vi "Clean Up Structures.vi"(8 "error in (no error)":errorcluster, 11 "Block Diagram in":refnum<class "Block Diagram.lvclass">) -> (0 "error out":errorcluster, 3 "Block Diagram out":refnum<class "Block Diagram.lvclass">)   [LabVIEW 2015, in "Block Diagram.lvclass"]
uses:
  Block Diagram.lvclass
  Block Diagram.lvclass/Block Diagram.ctl
  Structures/Structures.lvclass
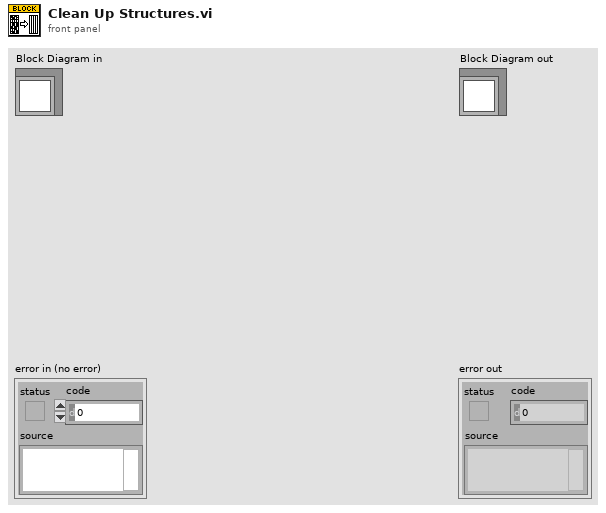
[diagram p1: front panel]
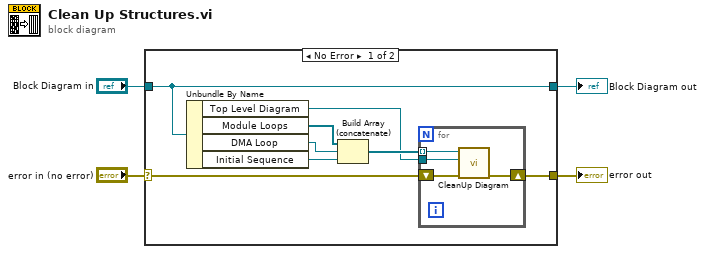
[diagram p0: block diagram]
diagram:
  n1 = case shown="No Error" "error in (no error)" {
    selector: "error in (no error)" -> [w11 w18]
    tunnel: [w5 w18] -> w3
    tunnel: [w12 w17] -> w1
    tunnel: "Block Diagram in" -> [w12 w17]
    frame No Error {
      n2 = Unbundle By Name(w12) -> ("Top Level Diagram"=w7:refnum<vi>, "Module Loops"=w9:refnum<class "Module Loop.lvclass">[], "DMA Loop"=w10:refnum<class "DMA Loop.lvclass">, "Initial Sequence"=w6:refnum<class "Main Sequence.lvclass">)
      n3 = Build Array (concatenate)(w9, w10, w6) -> (w8:refnum<class "Structures.lvclass">[])
      n4 = for {
        tunnel: w8 -> [w16] mode=indexing
        tunnel: w7 -> [w15]
        shift-right: [w13] -> w5
        shift-left: w11 -> [w14]
        n5 = call-dynamic "CleanUp Diagram.vi"("error in (no error)"=w14, "Top Level Diagram"=w15, "Structures in"=w16) -> ("error out"=w13:errorcluster)  [unwired: 7 in, 1 out]
      }
    }
    frame Error {
    }
  }
  "error out" <- w3
  "Block Diagram out" <- w1
